vi "prova a scrivere var da file ini.vi"   [LabVIEW 2020]
uses:
  NI9205/TYPEDEF/NI9205_TD_Method.ctl
types:
  T1 = typedef "_DRIVER_SHARED_TYPEDEF_StringControlVaviables.ctl" = cluster{"Ctrl Var Name":string, "String Ctrl Var Value":string}
  T2 = typedef "NI9205_TD_Method.ctl" = enum16{"NO_OP", "INIT", "SET", "GET", "CLOSE"}
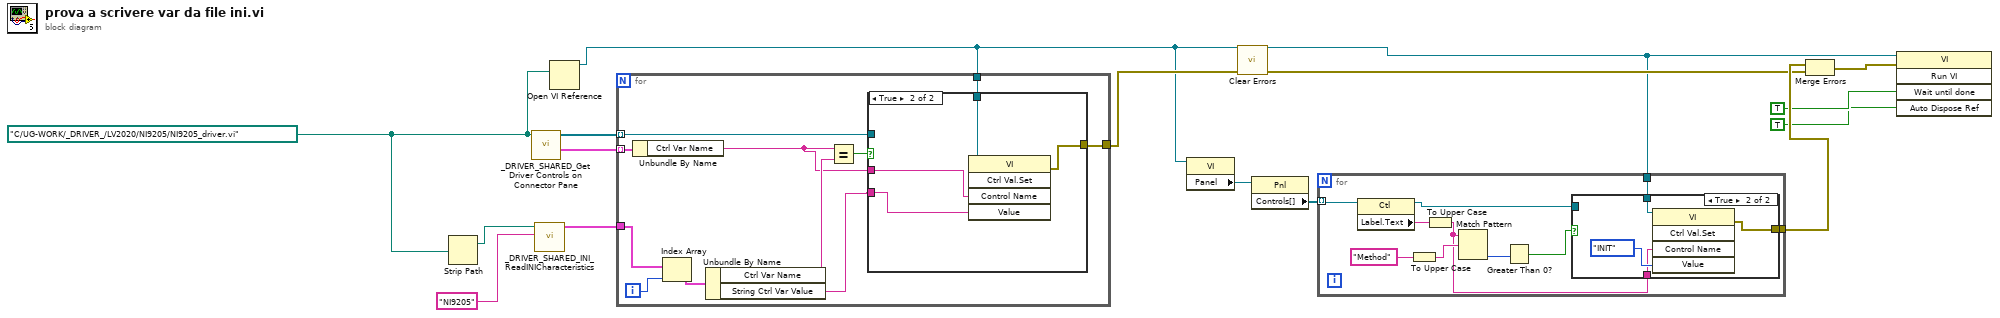
[diagram p0: block diagram]
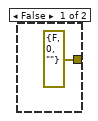
[diagram p2: hidden frame]
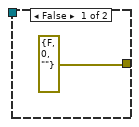
[diagram p3: hidden frame]
diagram:
  w1 = path "C:/UG-WORK/_DRIVER_/LV2020/NI9205/NI9205_driver.vi" ("Path of [...]_driver.vi")
  n1 = Strip Path(path=w1) -> (stripped path=w15:path)  [unwired: 1 out]
  n2 = call "_DRIVER_SHARED_Get Driver Controls on Connector Pane.vi"("Path of [...]_driver.vi"=w1) -> ("String Control Variables"=w12:T1[], "Ctrls ref"=w11:refnum<vi>[])  [unwired: 6 in, 3 out]
  n3 = call "_DRIVER_SHARED_INI_ReadINICharacteristics.vi"("Driver to Sel"="NI9205", "Path of \"_HW-Configuration_.ini\""=w15) -> ("INPUT Values"=w13:T1[])  [unwired: 8 in, 1 out]
  n4 = Open VI Reference(vi path=w1) -> (vi reference=w2:refnum<vi>)  [unwired: 5 in, 1 out]
  n5 = for {
    tunnel: w13 -> [w25]
    tunnel: w12 -> [w24] mode=indexing
    tunnel: w11 -> [w19] mode=indexing
    tunnel: [w18] -> w4
    tunnel: w2 -> [w17]
    i -> [w26]
    n6 = Unbundle By Name(w24) -> ("Ctrl Var Name"=w16:string)
    n7 = Index Array(array=w25, index=w26) -> (element=w22:T1)
    n8 = Unbundle By Name(w22) -> ("Ctrl Var Name"=w21:string, "String Ctrl Var Value"=w20:string)
    n9 = Equal?(x=w16, y=w21) -> (x = y?=w23:bool)
    n10 = case shown="True" w23 {
      tunnel: w20 -> [_ w29]
      tunnel: w19 -> [_ _]
      tunnel: [errorcluster {"status"=FALSE, "code"=0, "source"=""} ("error out") w28] -> w18
      tunnel: w17 -> [_ w31]
      tunnel: w16 -> [_ w30]
      frame False {
      }
      frame True {
        n11 = invoke class="VI" method="Ctrl Val.Set"(reference=w31, "Control Name"=w30, "Value"=w29) -> (error out=w28:errorcluster)  [unwired: 2 in, 4 out]
      }
    }
  }
  n12 = property class="VI"(reference=w2) -> ("Panel"=w10:refnum<vi>)  [unwired: 1 in, 2 out]
  n13 = call <vilib>:"Clear Errors.vi"("error in (no error)"=w4) -> ("error out"=w3:errorcluster)  [unwired: 5 in, 1 out]
  n14 = property class="Pnl"(reference=w10) -> ("Controls[]"=w9:refnum<vi>[])  [unwired: 1 in, 2 out]
  n15 = for {
    tunnel: w9 -> [w41] mode=indexing
    tunnel: [w34] -> w8
    tunnel: w2 -> [w33]
    n16 = property class="Ctl"(reference=w41) -> (reference out=w36:refnum<vi>, "Label.Text"=w40:string)  [unwired: 1 in, 1 out]
    n17 = To Upper Case(1:"Method" ("string")) -> (0:w39:string)
    n18 = To Upper Case(1:w40) -> (0:w32:string)
    n19 = Match Pattern(string=w32, regular expression=w39) -> (offset past match=w37:i32)  [unwired: 1 in, 3 out]
    n20 = Greater Than 0?(x=w37) -> (x > 0?=w35:bool)
    n21 = case shown="True" w35 {
      tunnel: w36 -> [_ _]
      tunnel: [errorcluster {"status"=FALSE, "code"=0, "source"=""} ("error out") w43] -> w34
      tunnel: w33 -> [_ w46]
      tunnel: w32 -> [_ w44]
      frame False {
      }
      frame True {
        n22 = invoke class="VI" method="Ctrl Val.Set"(reference=w46, "Control Name"=w44, "Value"=NI9205_TD_Method."INIT" ("Method NI9205")) -> (error out=w43:errorcluster)  [unwired: 2 in, 4 out]
      }
    }
  }
  n23 = Merge Errors(w8, w3) -> (w5:errorcluster)
  n24 = invoke class="VI" method="Run VI"(reference=w2, error in=w5, "Wait until done"=TRUE ("Wait Until Done"), "Auto Dispose Ref"=TRUE ("Auto Dispose Reference")) -> ()  [unwired: 1 in, 5 out]
